vi "dfd_Check Rational Factor.vi"(8 "error in (no error)":errorcluster, 11 "rational factor in":T1) -> (0 "error out":errorcluster, 1 "M":i32, 2 "L":i32, 3 "rational factor out":T1)   [LabVIEW 2017, in "NI_DigFilterLicensed.lvlib"]
uses:
  <vilib>/addons/Digital Filter Design/NI_DigFilterLicensed.lvlib
  <vilib>/addons/Digital Filter Design/_Objects.llb/DFD Multirate Rational Factor.ctl
  <vilib>/addons/Digital Filter Design/_Misc.llb/dfd_Error Handlers (Multiple).vi
  <vilib>/gmath/NI_Gmath.lvlib
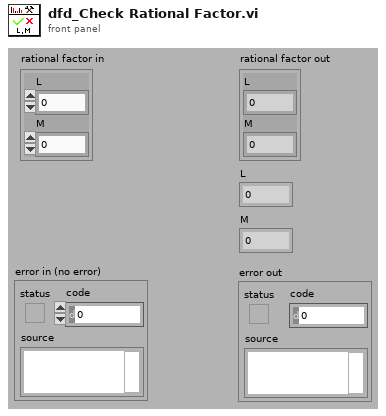
[diagram p1: front panel]
types:
  T1 = typedef "NI_DigFilterLicensed.lvlib/DFD Multirate Rational Factor.ctl" = cluster{"L":i32, "M":i32}
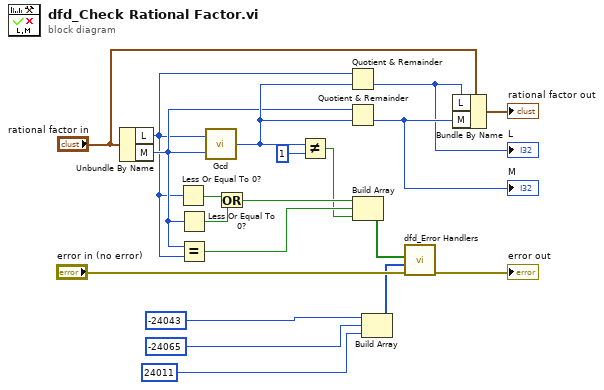
[diagram p0: block diagram]
diagram:
  n1 = Unbundle By Name("rational factor in") -> ("L"=w7:i32, "M"=w8:i32)
  n2 = Less Or Equal To 0?(x=w7) -> (x <= 0?=w20:bool)
  n3 = Less Or Equal To 0?(x=w8) -> (x <= 0?=w10:bool)
  n4 = Equal?(x=w8, y=w7) -> (x = y?=w6:bool)
  n5 = call <vilib>:"Gcd.vi"("y"=w8, "x"=w7) -> ("gcd(x,y)"=w13:i32)
  n6 = Or(x=w20, y=w10) -> (x .or. y?=w15:bool)
  n7 = Not Equal?(x=w13, y=1) -> (x != y?=w1:bool)
  n8 = Quotient & Remainder(x=w7, y=w13) -> (floor(x/y)=w3:i32)  [unwired: 1 out]
  "L" <- w3
  n9 = Quotient & Remainder(x=w8, y=w13) -> (floor(x/y)=w11:i32)  [unwired: 1 out]
  "M" <- w11
  n10 = Build Array(w15, w6, w1) -> (w16:bool[])
  n11 = Build Array(-24043 ("ERR_FACTOR_LE_ZERO"), -24065 ("ERR_L_M_EQUAL"), 24011 ("WRN_FACTOR_NOT_COPRIME")) -> (w14:i32[])
  n12 = call-poly <vilib>:"dfd_Error Handlers.vi"("error in (no error)"="error in (no error)", "error sources"=w14, "condition failed?"=w16) -> ("error out"=→"error out":errorcluster)  [unwired: 8 out]
  n13 = Bundle By Name(cluster="rational factor in", "L"=w3, "M"=w11) -> (→"rational factor out":T1)
